vi "phase_analysis.vi"(6 "data":waveform(dbl)[](array[waveform]), 9 "Channel in":T2 items=["Vin", "Woofer", "Tweeter", "Midrange"], 10 "Array in":T1(array[cluster]), 11 "Analizza F":bool) -> (3 "Array out":T1(array[cluster]))   [LabVIEW 2023]
uses:
  <vilib>/measure/NI_MAPro.lvlib
  <vilib>/measure/matone.llb/Extract Single Tone Information 1 Chan.vi
  Channel_choiche.ctl
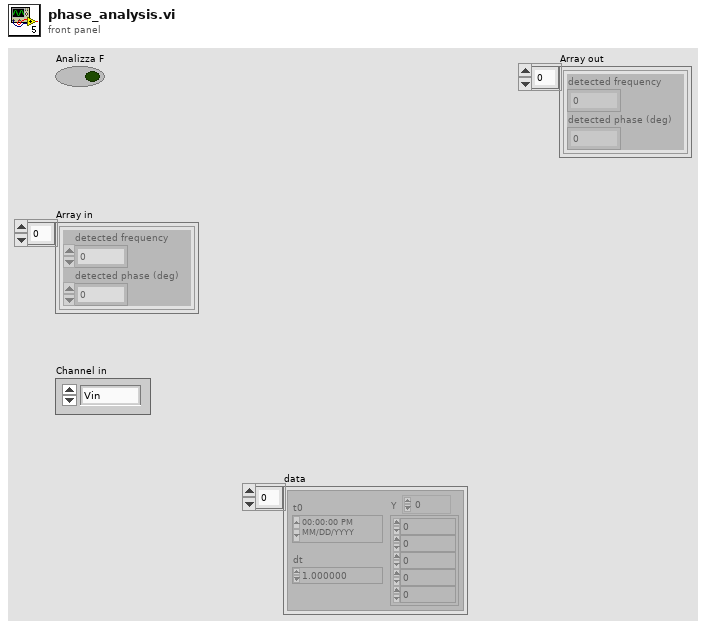
[diagram p1: front panel]
types:
  T1 = cluster{"detected frequency":dbl, "detected phase (deg)":dbl}[]
  T2 = typedef "Channel_choiche.ctl" = i16
  T3 = cluster{"detected frequency":dbl, "detected phase (deg)":dbl}
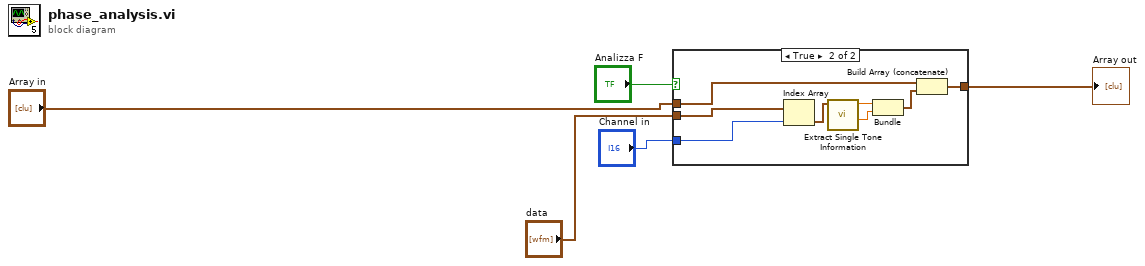
[diagram p0: block diagram]
diagram:
  n1 = case shown="True" "Analizza F" {
    tunnel: "data" -> [_ w13]
    tunnel: "Array in" -> [w6 w14]
    tunnel: [w6 w9] -> w4
    tunnel: "Channel in" -> [_ w7]
    frame False {
    }
    frame True {
      n2 = Index Array(array=w13, index=w7) -> (element=w12:waveform(dbl))
      n3 = call-poly <vilib>:"Extract Single Tone Information.vi"("time signal in"=w12) -> ("detected phase (deg)"=w10:dbl, "detected frequency"=w11:dbl)  [unwired: 5 in, 4 out]
      n4 = Bundle("detected frequency"=w11, "detected phase (deg)"=w10) -> (w8:T3)  [unwired: 1 in]
      n5 = Build Array (concatenate)(w14, w8) -> (w9:T1)
    }
  }
  "Array out" <- w4
